vi "Control, Hide and Move.vi"(4 "Y (0)":i32, 5 "X (0)":i32, 6 "error in":errorcluster, 9 "Ctl ref":refnum<vi>) -> (0 "error out":errorcluster, 3 "Ctl ref dup":refnum<vi>)   [LabVIEW 2010]
doc: "This function hides a control and moves it to the origin position (default)."
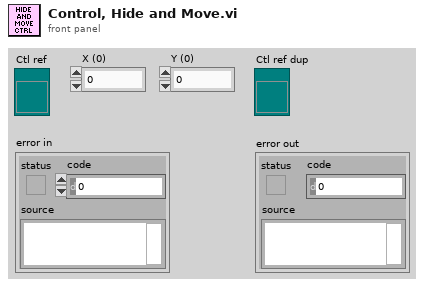
[diagram p1: front panel]
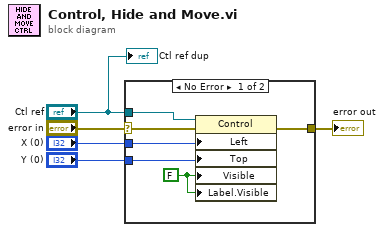
[diagram p0: block diagram]
diagram:
  n1 = case shown="No Error" "error in" {
    selector: "error in" -> [w10 w12]
    tunnel: [w9 w12] -> w5
    tunnel: "Ctl ref" -> [w11 _]
    tunnel: "X (0)" -> [w7 _]
    tunnel: "Y (0)" -> [w6 _]
    frame No Error {
      w8 = FALSE ("Visible")
      n2 = property class="Control"(reference=w11, error in=w10, "Left"=w7, "Top"=w6, "Visible"=w8, "Label.Visible"=w8) -> (error out=w9:errorcluster)  [unwired: 1 out]
    }
    frame Error {
    }
  }
  "error out" <- w5
  "Ctl ref dup" <- "Ctl ref"
